vi "OpenTestImage.vi"() -> ()   [LabVIEW 2011]
uses:
  <vilib>/Utility/miscctls.llb/LVPositionTypeDef.ctl
  CudaImage.ctl
  cudatrack-debug.dll
panel:
  out "Original 2":T1(plugin-control)
  out "Position":T2
  out "Cluster 2":cluster{"comX":sgl, "comY":sgl}
  out "Original":T1(plugin-control)
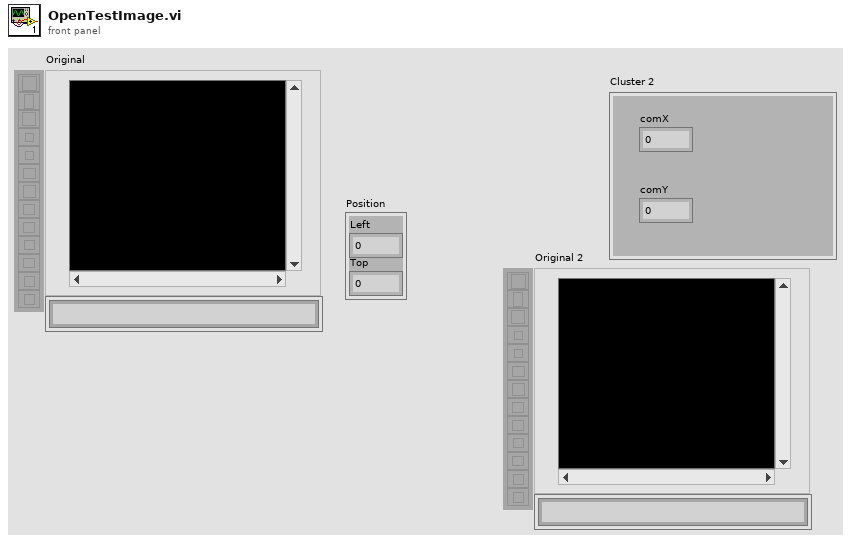
[diagram p1: front panel]
types:
  T1 = typedef "IMAQ Image.ctl" = refnum<image>
  T2 = typedef "LVPositionTypeDef.ctl" = cluster{"Left":i32, "Top":i32}
  T3 = typedef "CudaImage.ctl" = u64
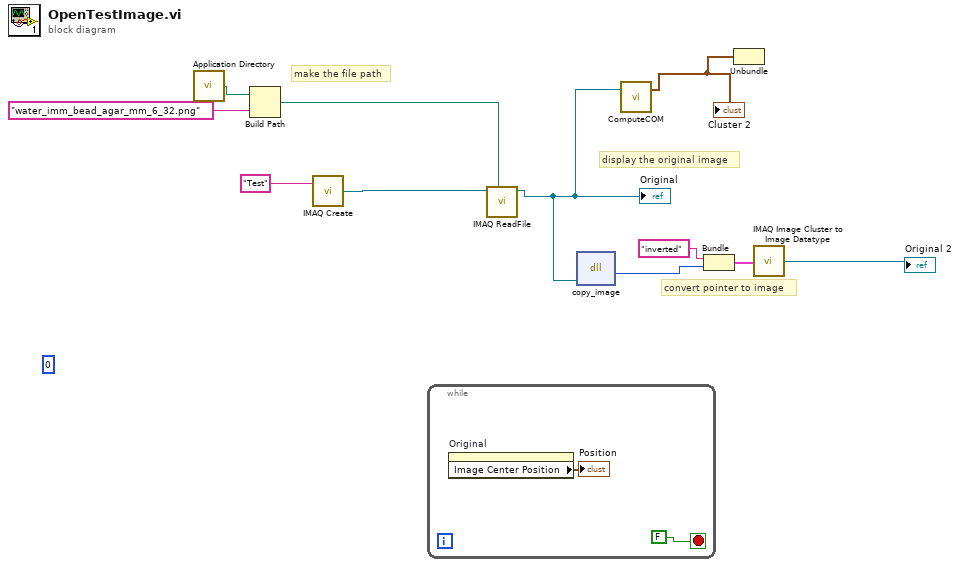
[diagram p0: block diagram]
diagram:
  (unwired) T3 0
  # "convert pointer to image"
  # "display the original image"
  # "make the file path"
  n1 = call <vilib>:"Application Directory.vi"() -> ("Application Directory"=w9:path)
  n2 = Build Path(base path=w9, name or relative path="water_imm_bead_agar_mm_6_32.png") -> (appended path=w7:path)
  n3 = call "IMAQ Create"("Image Name"="Test" ("String")) -> ("New Image"=w10:T1)  [unwired: 4 in, 1 out]
  n4 = while {
    stop <- FALSE stop-if-true
    n5 = property on="Original" class="ImageControl"() -> ("Image Center Position"=→"Position":cluster{"X":u32, "Y":u32})  [unwired: 2 in, 2 out]
  }
  n6 = call "IMAQ ReadFile"("File Path"=w7, "Image"=w10) -> ("Image Out"=w5:T1)  [unwired: 5 in, 4 out]
  "Original" <- w5
  n7 = dll-call lib="D:/jcnossen1/cudaqi-tracker/cudaqi/cudatrack-debug.dll" fn="copy_image"("srcImage"=w5) -> ("return type"=w3:u64)  [unwired: 4 in, 2 out]
  n8 = call "ComputeCOM.vi"("Image"=w5) -> ("Cluster 2"=w6:cluster{"comX":sgl, "comY":sgl})  [unwired: 2 in]
  "Cluster 2" <- w6
  n9 = Bundle("inverted", "return type"=w3) -> (w1:cluster{string, "return type":u64})  [unwired: 1 in]
  n10 = Unbundle(w6) -> ()  [unwired: 2 out]
  n11 = call <vilib>:"IMAQ Image Cluster to Image Datatype.vi"("Image"=w1) -> ("Image (dup)"=→"Original 2":T1)
